vi "DN4_DI_RegisterEvent.vi"(2 "DI Interrupt":refnum<user-event>, 3 "Task ID":u32) -> (0 "DI Interrupt":refnum<user-event>)   [LabVIEW 2009]
uses:
  Windows/System32/AdvLvDaq.dll
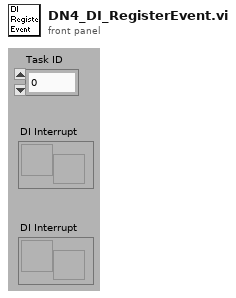
[diagram p1: front panel]
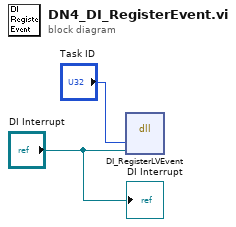
[diagram p0: block diagram]
diagram:
  n1 = dll-call lib="C:/Windows/System32/AdvLvDaq.dll" fn="DI_RegisterLVEvent"("taskId"="Task ID", "diSnap"="DI Interrupt") -> ()  [unwired: 4 in, 4 out]
  "DI Interrupt" <- "DI Interrupt"
